vi "noColisionManMarkerWithCenterBack.vi"(8 "error in (no error)":errorcluster, 9 "Pos ManMarker 2":dbl[](array[numeric]) format="%#_13g", 10 "Pos CenterBacks":dbl[][](array[numeric]) format="%#_13g", 11 "Utilities in":refnum<class "Utilities.lvclass">) -> (0 "error out":errorcluster, 2 "Pos ManMarker":dbl[](array[numeric]) format="%#_13g", 3 "Utilities out":refnum<class "Utilities.lvclass">)   [LabVIEW 2020, in "Utilities.lvclass"]
uses:
  Utilities.lvclass
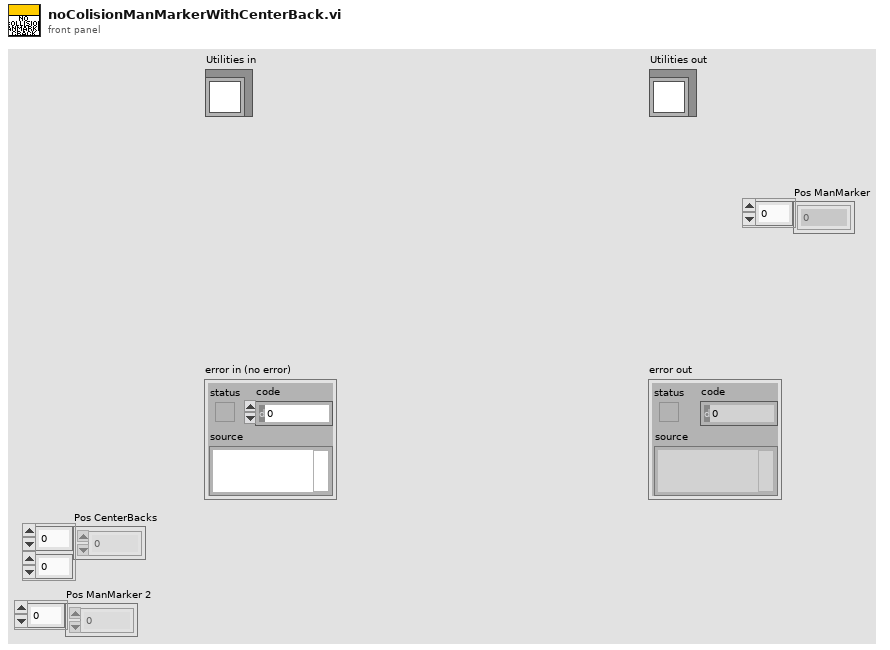
[diagram p1: front panel]
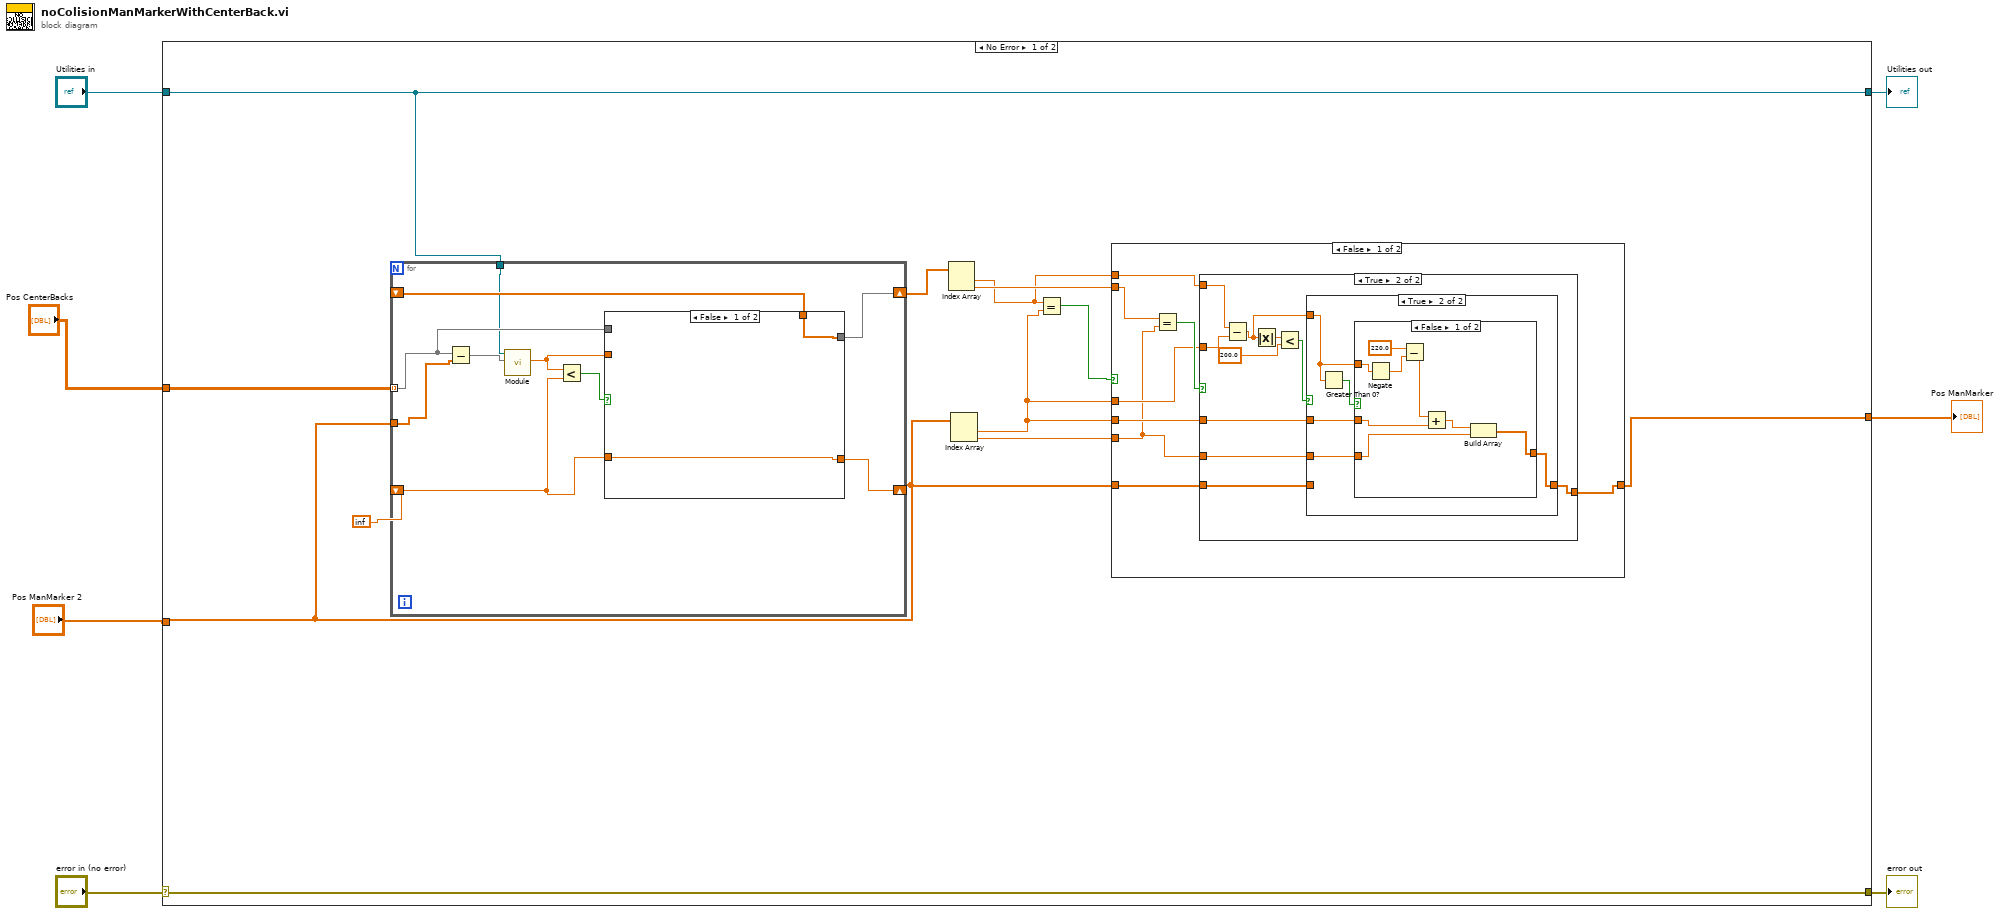
[diagram p0: block diagram]
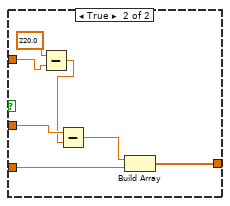
[diagram p4: hidden frame]
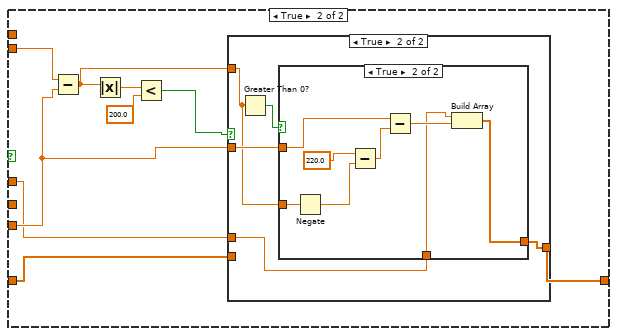
[diagram p5: hidden frame]
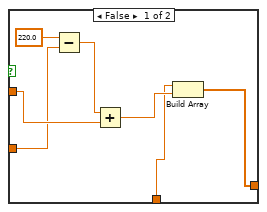
[diagram p7: hidden frame]
diagram:
  n1 = case shown="No Error" "error in (no error)" {
    selector: "error in (no error)" -> [w19 w105]
    tunnel: [w19 w105] -> w6
    tunnel: [w8 w104] -> w4
    tunnel: "Utilities in" -> [w8 w104]
    tunnel: "Pos ManMarker 2" -> [w11 _]
    tunnel: "Pos CenterBacks" -> [w10 _]
    tunnel: [w9 _] -> w1
    frame No Error {
      n2 = for {
        tunnel: w10 -> [w95] mode=indexing
        tunnel: w11 -> [w99]
        shift-right: [w97] -> _
        shift-left: inf -> [w93]
        shift-right: [w96] -> w17
        shift-left: _ -> [w94]
        tunnel: w8 -> [w90]
        n3 = Subtract(x=w95, y=w99) -> (x-y=w92:dbl[])
        n4 = call-dynamic "Module.vi"("2D vector"=w92, "Utilities in"=w90) -> ("Modulo"=w91:dbl)  [unwired: 7 in, 2 out]
        n5 = Less?(x=w91, y=w93) -> (x < y?=w98:bool)
        n6 = case shown="False" w98 {
          tunnel: [w101 w103] -> w97
          tunnel: w91 -> [_ w103]
          tunnel: w93 -> [w101 _]
          tunnel: [w100 w102] -> w96
          tunnel: w95 -> [_ w102]
          tunnel: w94 -> [w100 _]
          frame False {
          }
          frame True {
          }
        }
      }
      n7 = Index Array(array=w17) -> (element #1=w13:dbl, element #2=w15:dbl)  [unwired: 2 in]
      n8 = Index Array(array=w11) -> (element #1=w12:dbl, element #2=w14:dbl)  [unwired: 2 in]
      n9 = Equal?(x=w13, y=w12) -> (x = y?=w16:bool)
      n10 = case shown="False" w16 {
        tunnel: w15 -> [w27 w68]
        tunnel: w14 -> [w20 w62]
        tunnel: [w25 w64] -> w9
        tunnel: w11 -> [w24 w63]
        tunnel: w12 -> [w22 w60]
        tunnel: w13 -> [w23 _]
        tunnel: w12 -> [w21 _]
        frame False {
          n11 = Equal?(x=w27, y=w20) -> (x = y?=w26:bool)
          n12 = case shown="True" w26 {
            tunnel: [w28 w34] -> w25
            tunnel: w24 -> [w28 w33]
            tunnel: w23 -> [_ w38]
            tunnel: w22 -> [_ w37]
            tunnel: w21 -> [_ w30]
            tunnel: w20 -> [_ w29]
            frame False {
            }
            frame True {
              n13 = Subtract(x=w38, y=w37) -> (x-y=w31:dbl)
              n14 = Absolute Value(x=w31) -> (abs(x)=w32:dbl)
              n15 = Less?(x=w32, y=200.0) -> (x < y?=w35:bool)
              n16 = case shown="True" w35 {
                tunnel: [w39 w41] -> w34
                tunnel: w33 -> [w39 _]
                tunnel: w31 -> [_ w42]
                tunnel: w30 -> [_ w43]
                tunnel: w29 -> [_ w40]
                frame False {
                }
                frame True {
                  n17 = Greater Than 0?(x=w42) -> (x > 0?=w44:bool)
                  n18 = case shown="False" w44 {
                    tunnel: w43 -> [w52 w59]
                    tunnel: w42 -> [w50 w57]
                    tunnel: [w47 w54] -> w41
                    tunnel: w40 -> [w45 w53]
                    frame False {
                      n19 = Negate(x=w50) -> (-x=w49:dbl)
                      n20 = Subtract(x=220.0, y=w49) -> (x-y=w48:dbl)
                      n21 = Add(x=w48, y=w52) -> (x+y=w46:dbl)
                      n22 = Build Array(w46, w45) -> (w47:dbl[])
                    }
                    frame True {
                      n23 = Subtract(x=220.0, y=w57) -> (x-y=w56:dbl)
                      n24 = Subtract(x=w59, y=w56) -> (x-y=w55:dbl)
                      n25 = Build Array(w55, w53) -> (w54:dbl[])
                    }
                  }
                }
              }
            }
          }
        }
        frame True {
          n26 = Subtract(x=w68, y=w62) -> (x-y=w61:dbl)
          n27 = Absolute Value(x=w61) -> (abs(x)=w67:dbl)
          n28 = Less?(x=w67, y=200.0) -> (x < y?=w65:bool)
          n29 = case shown="True" w65 {
            tunnel: [w69 w71] -> w64
            tunnel: w63 -> [w69 _]
            tunnel: w61 -> [_ w70]
            tunnel: w62 -> [_ w73]
            tunnel: w60 -> [_ w72]
            frame False {
            }
            frame True {
              n30 = Greater Than 0?(x=w70) -> (x > 0?=w74:bool)
              n31 = case shown="True" w74 {
                tunnel: w73 -> [w81 w89]
                tunnel: w70 -> [w79 w83]
                tunnel: w72 -> [w76 w85]
                tunnel: [w75 w84] -> w71
                frame False {
                  n32 = Subtract(x=220.0, y=w79) -> (x-y=w78:dbl)
                  n33 = Add(x=w78, y=w81) -> (x+y=w77:dbl)
                  n34 = Build Array(w76, w77) -> (w75:dbl[])
                }
                frame True {
                  n35 = Negate(x=w83) -> (-x=w82:dbl)
                  n36 = Subtract(x=220.0, y=w82) -> (x-y=w87:dbl)
                  n37 = Subtract(x=w89, y=w87) -> (x-y=w86:dbl)
                  n38 = Build Array(w85, w86) -> (w84:dbl[])
                }
              }
            }
          }
        }
      }
    }
    frame Error {
    }
  }
  "error out" <- w6
  "Utilities out" <- w4
  "Pos ManMarker" <- w1
